vi "Ping_Dead.vi"(0 "ModelNumber":string, 1 "error in":errorcluster caption="错误输入（无错误）") -> (2 "Acess":bool, 3 "standard output":string caption="标准输出", 4 "error out":errorcluster caption="错误输出")   [LabVIEW 2013]
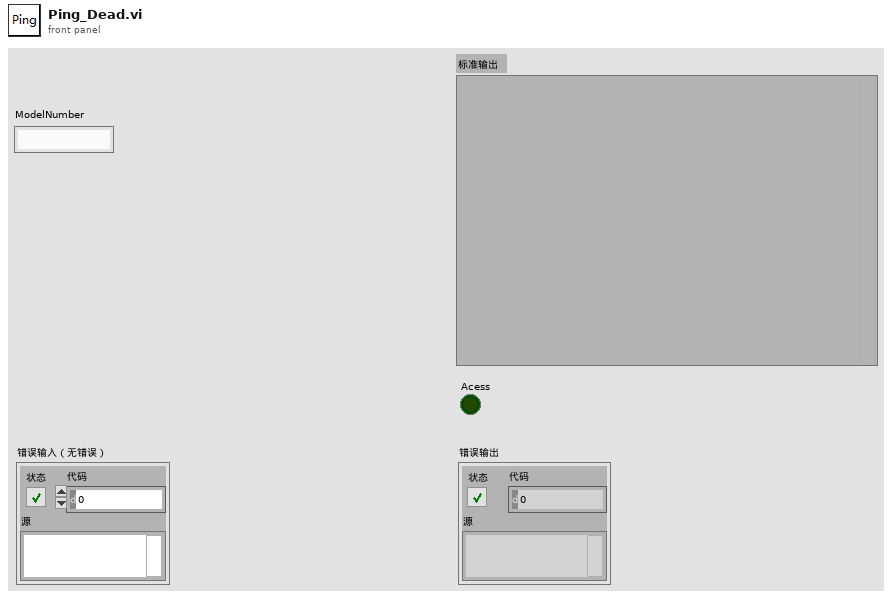
[diagram p1: front panel]
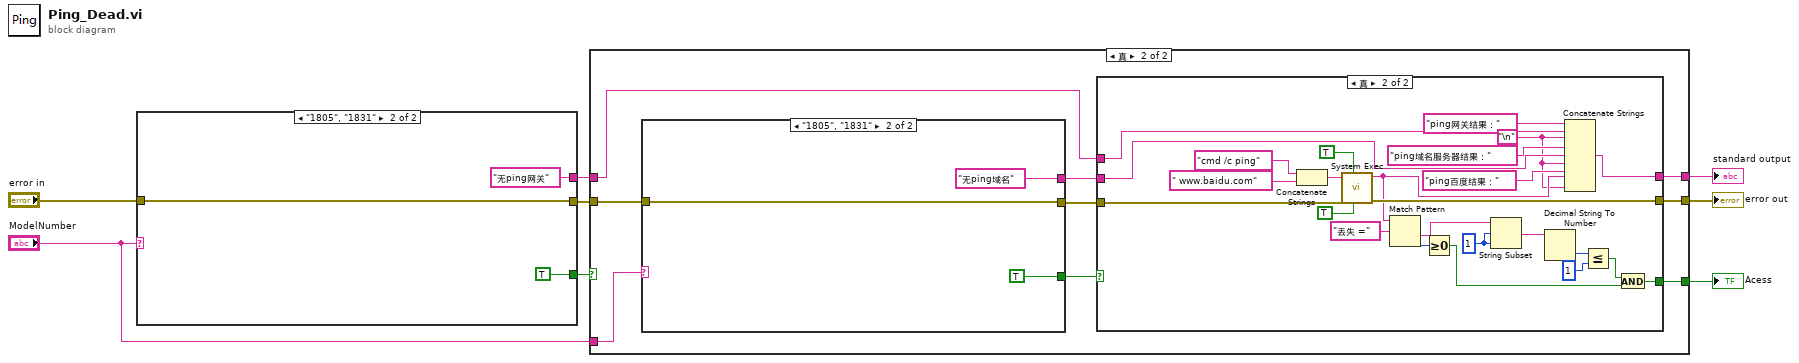
[diagram p0: block diagram]
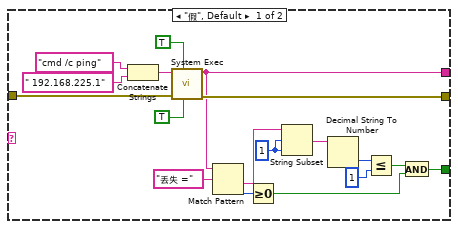
[diagram p2: hidden frame]
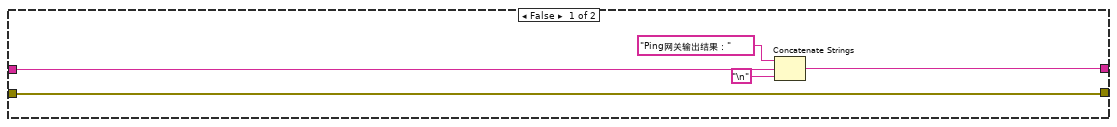
[diagram p3: hidden frame]
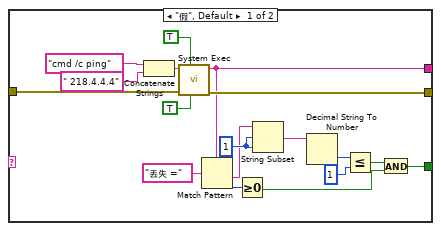
[diagram p4: hidden frame]
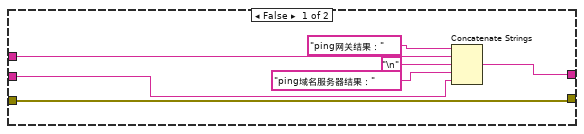
[diagram p5: hidden frame]
diagram:
  n1 = case shown="\"1805\", \"1831\"" "ModelNumber" {
    tunnel: "error in" -> [w26 w28]
    tunnel: [w13 w28] -> w5
    tunnel: [w12 TRUE ("run minimized? (F)")] -> w4
    tunnel: [w11 "无ping网关" ("standard output")] -> w2
    frame "假", Default {
      w19 = 1
      n2 = Concatenate Strings("cmd /c ping" ("command line"), " 192.168.225.1" ("Adress")) -> (w23:string)
      n3 = call <vilib>:"System Exec.vi"("run minimized? (F)"=TRUE, "wait until completion? (T)"=TRUE ("run minimized? (F)"), "error in (no error)"=w26, "command line"=w23) -> ("error out"=w13:errorcluster, "standard output"=w11:string)  [unwired: 4 in, 2 out]
      n4 = Match Pattern(string=w11, regular expression="丢失 =" ("正则表达式")) -> (after substring=w18:string, offset past match=w17:i32)  [unwired: 1 in, 2 out]
      n5 = Greater Or Equal To 0?(x=w17) -> (x >= 0?=w14:bool)
      n6 = String Subset(string=w18, offset (0)=w19, length (rest)=w19) -> (substring=w20:string)
      n7 = Decimal String To Number(string=w20) -> (number=w21:i32)  [unwired: 2 in, 1 out]
      n8 = Less Or Equal?(x=w21, y=1) -> (x <= y?=w15:bool)
      n9 = And(x=w15, y=w14) -> (x .and. y?=w12:bool)
    }
    frame "1805", "1831" {
    }
  }
  n10 = case shown="真" w4 {
    tunnel: [_ w43] -> w8
    tunnel: [w34 w42] -> w7
    tunnel: w5 -> [w34 w41]
    tunnel: [w33 w39] -> w3
    tunnel: w2 -> [w31 w37]
    tunnel: "ModelNumber" -> [_ w35]
    frame False {
      n11 = Concatenate Strings("Ping网关输出结果：", w31, "\n") -> (w33:string)
    }
    frame True {
      n12 = case shown="\"1805\", \"1831\"" w35 {
        tunnel: w41 -> [w59 w64]
        tunnel: [w57 w64] -> w40
        tunnel: [w48 TRUE ("run minimized? (F)")] -> w38
        tunnel: [w47 "无ping域名" ("standard output")] -> w36
        frame "假", Default {
          w52 = 1
          n13 = Concatenate Strings("cmd /c ping" ("command line"), " 218.4.4.4" ("Adress")) -> (w58:string)
          n14 = call <vilib>:"System Exec.vi"("run minimized? (F)"=TRUE, "wait until completion? (T)"=TRUE ("run minimized? (F)"), "error in (no error)"=w59, "command line"=w58) -> ("error out"=w57:errorcluster, "standard output"=w47:string)  [unwired: 4 in, 2 out]
          n15 = Match Pattern(string=w47, regular expression="丢失 =" ("正则表达式")) -> (after substring=w46:string, offset past match=w53:i32)  [unwired: 1 in, 2 out]
          n16 = Greater Or Equal To 0?(x=w53) -> (x >= 0?=w56:bool)
          n17 = String Subset(string=w46, offset (0)=w52, length (rest)=w52) -> (substring=w51:string)
          n18 = Decimal String To Number(string=w51) -> (number=w50:i32)  [unwired: 2 in, 1 out]
          n19 = Less Or Equal?(x=w50, y=1) -> (x <= y?=w55:bool)
          n20 = And(x=w55, y=w56) -> (x .and. y?=w48:bool)
        }
        frame "1805", "1831" {
        }
      }
      n21 = case shown="真" w38 {
        tunnel: [_ w86] -> w43
        tunnel: [w65 w85] -> w42
        tunnel: w40 -> [w65 w81]
        tunnel: [w66 w73] -> w39
        tunnel: w37 -> [w70 w79]
        tunnel: w36 -> [w67 w77]
        frame False {
          n22 = Concatenate Strings("ping网关结果：" ("command line"), w70, "\n", "ping域名服务器结果：" ("command line"), w67) -> (w66:string)
        }
        frame True {
          w74 = "\n"
          w92 = 1
          n23 = Concatenate Strings("cmd /c ping" ("command line"), " www.baidu.com" ("Adress")) -> (w84:string)
          n24 = call <vilib>:"System Exec.vi"("run minimized? (F)"=TRUE, "wait until completion? (T)"=TRUE ("run minimized? (F)"), "error in (no error)"=w81, "command line"=w84) -> ("error out"=w85:errorcluster, "standard output"=w75:string)  [unwired: 4 in, 2 out]
          n25 = Match Pattern(string=w75, regular expression="丢失 =" ("正则表达式")) -> (after substring=w93:string, offset past match=w94:i32)  [unwired: 1 in, 2 out]
          n26 = Greater Or Equal To 0?(x=w94) -> (x >= 0?=w87:bool)
          n27 = String Subset(string=w93, offset (0)=w92, length (rest)=w92) -> (substring=w91:string)
          n28 = Decimal String To Number(string=w91) -> (number=w90:i32)  [unwired: 2 in, 1 out]
          n29 = Concatenate Strings("ping网关结果：" ("command line"), w79, w74, "ping域名服务器结果：" ("command line"), w77, w74, "ping百度结果：" ("command line"), w75, w74) -> (w73:string)
          n30 = Less Or Equal?(x=w90, y=1) -> (x <= y?=w88:bool)
          n31 = And(x=w88, y=w87) -> (x .and. y?=w86:bool)
        }
      }
    }
  }
  "error out" <- w7
  "Acess" <- w8
  "standard output" <- w3
